vi "Get Impedance Meas Value.vi"(8 "error in (no error)":errorcluster, 11 "VISA resource name":refnum<visa-resource-name>) -> (0 "error out":errorcluster, 1 "Value Units":i32, 2 "Meas Value":dbl format="%^.3e", 3 "VISA resource name out":refnum<visa-resource-name>)   [LabVIEW 2014, in "Fluke 5XXX Series Multicalibrators.lvlib"]
doc: "This VI returns the last value of the scope impedance measurement. The unit returns indicates the status of the reading. Returns 0 and NONE when there is no recent measurement either because the Calibrator is not in a measurement mode, or because no measurement has been made yet.\n\nNote:\n\nThis VI is available only for instrument models 5500A and 5520A with oscilloscope option SC600 (SC1100)."
uses:
  Fluke 5XXX Series Multicalibrators.lvlib
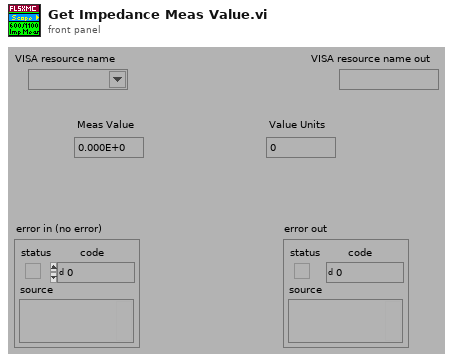
[diagram p1: front panel]
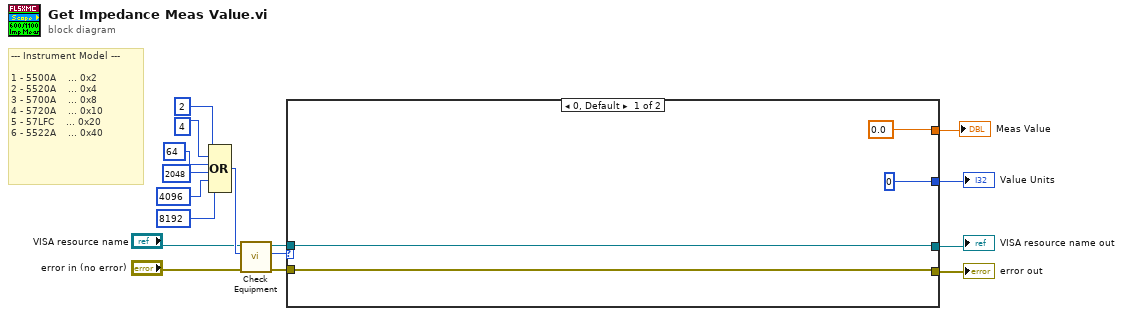
[diagram p0: block diagram]
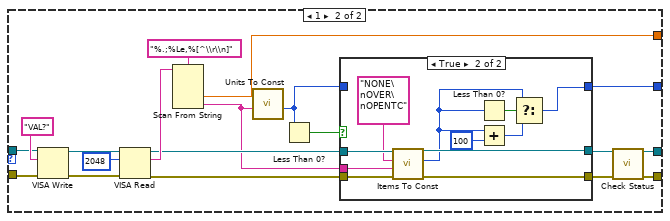
[diagram p2: hidden frame]
diagram:
  # "--- Instrument Model ---\n\n1 - 5500A    ... 0x2\n2 - 5520A    ... 0x4\n3 - 5700A    ... 0x8\n4 - 5720A    ... 0x10\n5 - 57LFC    ... 0x20\n6 - 5522A    ... 0x40"
  n1 = Compound Arithmetic op=OR(2 ("Numeric"), 4 ("Numeric"), 64 ("Numeric"), 2048 ("Numeric"), 4096 ("Numeric"), 8192 ("Numeric")) -> (w12:i32)
  n2 = call "Check Equipment.vi"("error in (no error)"="error in (no error)", "Bit Mask"=w12, "VISA resource name"="VISA resource name") -> ("error out"=w8:errorcluster, "Present?"=w7:u32, "VISA resource name out"=w9:refnum<visa-resource-name>)  [unwired: 6 in]
  n3 = case shown="0, Default" w7 {
    tunnel: [w20 w34] -> w5
    tunnel: [w17 w33] -> w6
    tunnel: w8 -> [w20 w35]
    tunnel: [0.0 w30] -> w3
    tunnel: [0 w28] -> w4
    tunnel: w9 -> [w17 w22]
    frame 0, Default {
    }
    frame 1 {
      n4 = VISA Write(VISA resource name=w22, write buffer="VAL?", error in (no error)=w35) -> (VISA resource name out=w38:refnum<visa-resource-name>, error out=w37:errorcluster)  [unwired: 1 out]
      n5 = VISA Read(VISA resource name=w38, byte count=u32 2048 ("byte count (0)"), error in (no error)=w37) -> (VISA resource name out=w27:refnum<visa-resource-name>, read buffer=w31:string, error out=w24:errorcluster)  [unwired: 1 out]
      n6 = Scan From String(format string="%.;%Le,%[^\\r\\n]", input string=w31) -> (output 1=w30:dbl, output 2=w23:string)  [unwired: 4 in, 3 out]
      n7 = call "Units To Const.vi"("Units"=w23) -> ("Const"=w21:i32)  [unwired: 10 in]
      n8 = Less Than 0?(x=w21) -> (x < 0?=w29:bool)
      n9 = case shown="True" w29 {
        tunnel: w21 -> [w42 _]
        tunnel: [w42 w49] -> w28
        tunnel: w27 -> [w40 w52]
        tunnel: [w40 w53] -> w26
        tunnel: [w41 w44] -> w25
        tunnel: w24 -> [w41 w46]
        tunnel: w23 -> [_ w50]
        frame False {
        }
        frame True {
          n10 = call "Items To Const.vi"("error in (no error)"=w46, "String Item"=w50, "Multi-Line String"="NONE\nOVER\nOPENTC", "VISA resource name"=w52) -> ("error out"=w44:errorcluster, "Index"=w43:i32, "VISA resource name out"=w53:refnum<visa-resource-name>)  [unwired: 5 in]
          n11 = Less Than 0?(x=w43) -> (x < 0?=w45:bool)
          n12 = Add(x=w43, y=100) -> (x+y=w48:i32)
          n13 = Select(t=w43, s=w45, f=w48) -> (s? t:f=w49:i32)
        }
      }
      n14 = call "Check Status.vi"("VISA resource name"=w26, "error in (no error)"=w25) -> ("VISA resource name out"=w33:refnum<visa-resource-name>, "error out"=w34:errorcluster)  [unwired: 12 in]
    }
  }
  "Meas Value" <- w3
  "Value Units" <- w4
  "VISA resource name out" <- w6
  "error out" <- w5
